vi "Init VMR API.vi"(8 "error in (no error)":errorcluster, 11 "VMR Server in":refnum<class "VMR Server.lvclass">) -> (0 "error out":errorcluster, 3 "VMR Server out":refnum<class "VMR Server.lvclass">)   [LabVIEW 2022 SP3, in "VMR Server.lvlib" / "VMR Server.lvclass"]
uses:
  VMR Server.lvclass
  VMR Server.lvclass/VMR Server.ctl
  <vilib>/ActorFramework/Actor/Actor.lvclass
  VMR Actor/VMR Actor.lvclass
  VMR Actor API/VMR Actor API.lvclass
  C:/Program Files (x86)/National Instruments/LabVIEW 2022/vi.lib/ActorFramework/Actor/Actor.lvclass
  C:/dev/lv/2022/touchcontrol/VMR Server/VMR Actor/VMR Actor.lvclass
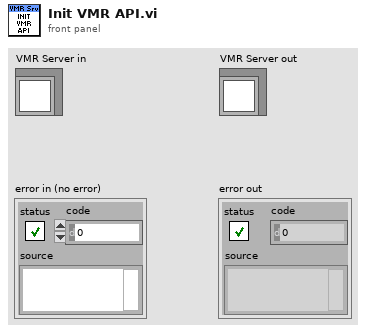
[diagram p1: front panel]
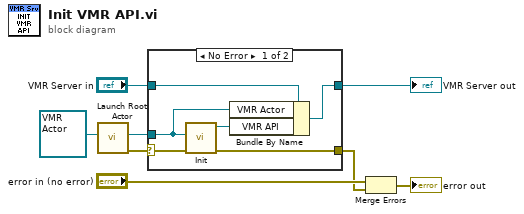
[diagram p0: block diagram]
diagram:
  n1 = call <vilib>:"Launch Root Actor.vi"("Actor"=refnum<class "VMR Actor.lvclass"> refnum ("VMR Server.lvlib:VMR Actor.lvclass")) -> ("error out"=w6:errorcluster, "Actor's Enqueuer"=w5:refnum<class "Message Enqueuer.lvclass">)  [unwired: 9 in]
  n2 = case shown="No Error" w6 {
    selector: w6 -> [w14 w15]
    tunnel: w5 -> [w13 _]
    tunnel: "VMR Server in" -> [w11 w16]
    tunnel: [w10 w16] -> w3
    tunnel: [w9 w15] -> w1
    frame No Error {
      n3 = call "Init.vi"("error in (no error)"=w14, "Enqueuer"=w13) -> ("error out"=w9:errorcluster, "VMR Actor API out"=w12:refnum<class "VMR Actor API.lvclass">)  [unwired: 8 in]
      n4 = Bundle By Name(cluster=w11, "VMR Actor"=w13, "VMR API"=w12) -> (w10:refnum<class "VMR Server.lvclass">)
    }
    frame Error {
    }
  }
  "VMR Server out" <- w3
  n5 = Merge Errors("error in (no error)", w1) -> (→"error out":errorcluster)
